vi "get_curr_position.vi"(8 "error in (no error)":errorcluster, 11 "ESP301viaTCPIP in":refnum<class "ESP301viaTCPIP.lvclass">) -> (0 "error out":errorcluster, 2 "readback position":dbl[](array[numeric]), 3 "ESP301viaTCPIP out":refnum<class "ESP301viaTCPIP.lvclass">)   [LabVIEW 2019, in "ESP301viaTCPIP.lvlib" / "ESP301viaTCPIP.lvclass"]
uses:
  ESP301viaTCPIP.lvclass
  _stage/_stage.lvlibp/_stageClass/_stage.lvclass
  ESP301viaTCPIP.lvlib
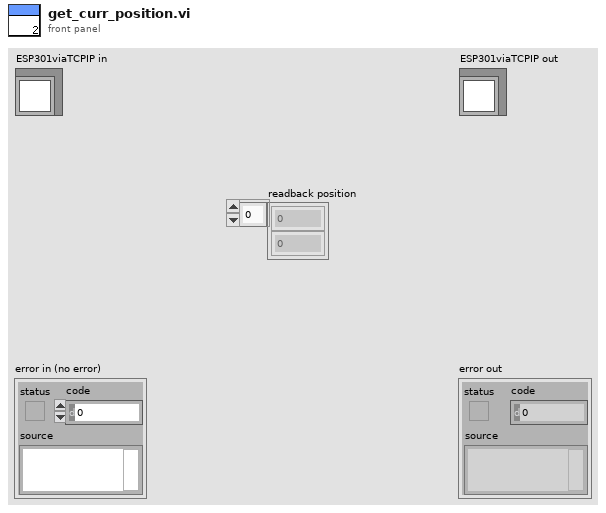
[diagram p1: front panel]
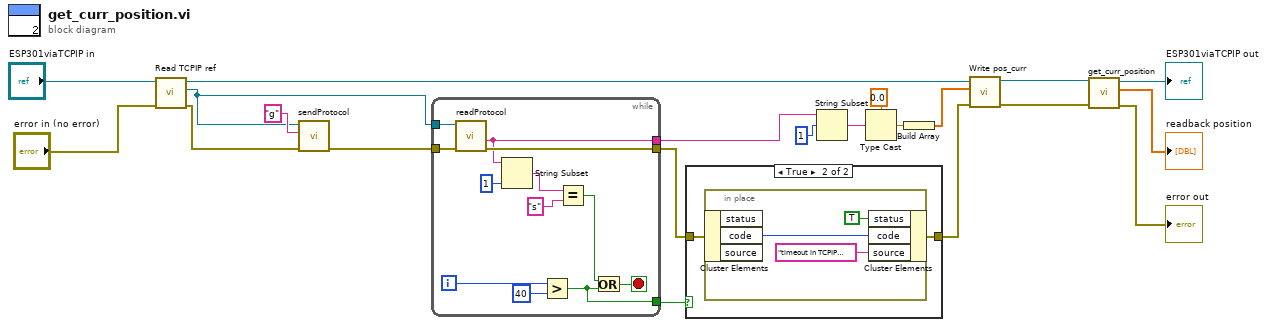
[diagram p0: block diagram]
diagram:
  n1 = call-dynamic "Read TCPIP ref.vi"("error in (no error)"="error in (no error)", "ESP301viaTCPIP in"="ESP301viaTCPIP in") -> ("error out"=w15:errorcluster, "TCPIP ref"=w6:refnum<k5>, "ESP301viaTCPIP out"=w4:refnum<class "ESP301viaTCPIP.lvclass">)  [unwired: 7 in]
  n2 = call "sendProtocol.vi"("error in (no error)"=w15, "command"="g", "TCP Network Connection in"=w6) -> ("error out"=w5:errorcluster)  [unwired: 7 in, 1 out]
  n3 = while {
    tunnel: w6 -> [w33]
    tunnel: w5 -> [w32]
    tunnel: [w28] -> w9
    tunnel: [w27] -> w14
    tunnel: [w22] -> w10
    i -> [w26]
    stop <- w23 stop-if-true
    n4 = call "readProtocol.vi"("error in (no error)"=w32, "TCP Network Connection in"=w33) -> ("error out"=w28:errorcluster, "data out"=w27:string)  [unwired: 8 in]
    n5 = String Subset(string=w27, length (rest)=1 ("length (rest)")) -> (substring=w30:string)  [unwired: 1 in]
    n6 = Greater?(x=w26, y=40) -> (0:w22:bool)
    n7 = Equal?(x=w30, y="s") -> (x = y?=w24:bool)
    n8 = Or(x=w24, y=w22) -> (x .or. y?=w23:bool)
  }
  n9 = case shown="True" w10 {
    tunnel: w9 -> [w34 w36]
    tunnel: [w34 w35] -> w8
    frame False {
    }
    frame True {
      n10 = in-place {
        n11 = in-place-cluster #1(w36) -> ("code"=w37:i32)  [unwired: 2 out]
        n12 = in-place-cluster #1("status"=TRUE, "code"=w37, "source"="timeout in TCPIP readback") -> (w35:errorcluster)
      }
    }
  }
  n13 = String Subset(string=w14, offset (0)=1 ("length (rest)")) -> (substring=w13:string)  [unwired: 1 in]
  n14 = Type Cast(type=0.0, x=w13) -> (*(type *) &x=w11:dbl)
  n15 = Build Array(w11) -> (w1:dbl[])
  n16 = call-dynamic "Write pos_curr.vi"("error in (no error)"=w8, "set_pos"=w1, "_stage in"=w4) -> ("error out"=w2:errorcluster, "_stage out"=w3:refnum<class "ESP301viaTCPIP.lvclass">)  [unwired: 7 in]
  n17 = call-parent "get_curr_position.vi"("error in (no error)"=w2, "_stage in"=w3) -> ("error out"=→"error out":errorcluster, "readback position"=→"readback position":dbl[], "_stage out"=→"ESP301viaTCPIP out":refnum<class "ESP301viaTCPIP.lvclass">)  [unwired: 7 in]
